vi "Validate live stimulus trig pulse width.vi"(9 "Requested trigger pulse width (ms)":dbl min=0.0 step=0.1, 11 "Trigger period (sec)":dbl) -> (2 "Live imaging. stimulus trigger pulse width (ms)":dbl format="%#_6f")   [LabVIEW 2017]
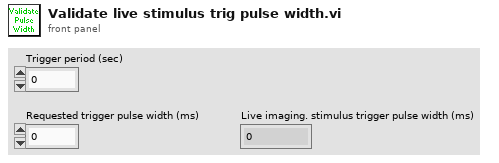
[diagram p1: front panel]
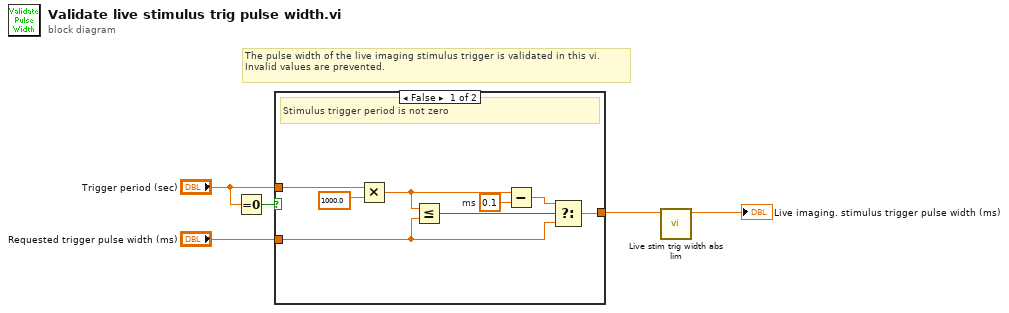
[diagram p0: block diagram]
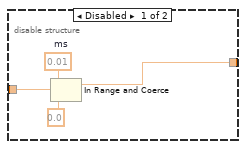
[diagram p3: hidden frame]
diagram:
  # "The pulse width of the live imaging stimulus trigger is validated in this vi.\nInvalid values are prevented."
  n1 = Equal To 0?(x="Trigger period (sec)") -> (x = 0?=w3:bool)
  n2 = case shown="False" w3 {
    tunnel: "Requested trigger pulse width (ms)" -> [w13 w15]
    tunnel: [w7 w14] -> w2
    tunnel: "Trigger period (sec)" -> [w6 _]
    frame False {
      w8 = 0.1  # ms
      # "Stimulus trigger period is not zero"
      n3 = Multiply(x=w6, y=1000.0) -> (x*y=w9:dbl)
      n4 = Less Or Equal?(x=w9, y=w13) -> (x <= y?=w11:bool)
      n5 = Subtract(x=w9, y=w8) -> (x-y=w12:dbl)
      n6 = Select(t=w12, s=w11, f=w13) -> (s? t:f=w7:dbl)
    }
    frame True {
      # "Stimulus trigger period is zero"
      n7 = disable-structure shown="Enabled" {
        disable-tunnel: w15 -> [w17 w20]
        disable-tunnel: [w16 w20] -> w14
        frame Disabled {
          w19 = 0.01  # ms
          n8 = In Range and Coerce(upper limit=w19, x=w17, lower limit=0.0) -> (coerced(x)=w16:dbl)  [unwired: 1 out]
        }
        frame Enabled {
        }
      }
    }
  }
  n9 = call "Live stim trig width abs lim.vi"("Live stim.trig.width (ms)"=w2) -> ("Live stim.trig.width (ms)"=→"Live imaging. stimulus trigger pulse width (ms)":dbl)  [unwired: 10 in]
